vi "Cepstrum Analysis.vi"() -> ()   [LabVIEW 2023]
doc: "This example shows how to compute the real cepstrum of a univariate time series with the TSA Real Cepstrum VI, to compute the complex cepstrum of a univariate time series with the TSA Complex Cepstrum VI, and to reconstruct original time series with the TSA Inverse Complex Cepstrum VI. \n\n<b>Instructions:</b>\n1) Run this VI.\n2) Observe the real and complex cepstrum with different settings."
uses:
  <vilib>/addons/Time Series Analysis/Utilities.llb/TSA Data.ctl
  <vilib>/addons/Time Series Analysis/Correlation and Spectral Analysis.llb/TSA Complex Cepstrum (Waveform).vi
  <vilib>/addons/Time Series Analysis/Correlation and Spectral Analysis.llb/TSA Inverse Complex Cepstrum (Waveform).vi
  <vilib>/addons/Time Series Analysis/Correlation and Spectral Analysis.llb/TSA Real Cepstrum (Waveform).vi
  <vilib>/addons/_Advanced Signal Processing/NI_AdvSigProcTSA.lvlib
panel:
  in  "stop":bool
  in  "AR setting":cluster{"Method":u16, "AR Order":i32}={"Method"=0, "AR Order"=60} {"Method" items=["Forward-Backward", "Least-Squares", "Yule-Walker", "Burg-Lattice", "Geometric-Lattice"]}
  in  "Cepstrum bins":i32=-1
  in  "Window":u16(ring) items=["None ", "Hanning", "Hamming", "Blackman-Harris", "Exact Blackman", "Blackman", "Flat Top", "4 Term B-Harris ", "7 Term B-Harris", "Low Sidelobe"]
  in  "Method for Real Cepstrum":u16(ring) items=["FFT", "AR Model"]
  out "Complex Cepstrum":cluster{"t0":dbl, "dt":dbl, "C(t)":dbl[]}(graph)
  out "Vibration Series":waveform(dbl)[](graph)
  out "Real Cepstrum":cluster{"t0":dbl, "dt":dbl, "C(t)":dbl[]}(graph)
  # "Overview: Shows how to compute the real cepstrum of a univariate time series with the TSA Real Cepstrum VI, to compute the complex cepstrum of a univariate time series with  the TSA Complex Cepstrum VI, and to reconstruct original time series with the TSA Inverse Complex Cepstrum VI.\nRequirements: LabVIEW Full Development System, Advanced Signal Processing Toolkit\nInstructions: \n1. Run this VI.\n2. Observe the real and complex cepstrum with different settings.\n3. Click Stop to stop the VI."
  # "Cepstrum Settings"
  # "Settings for the FFT Method"
  # "Settings for the AR Model Method"
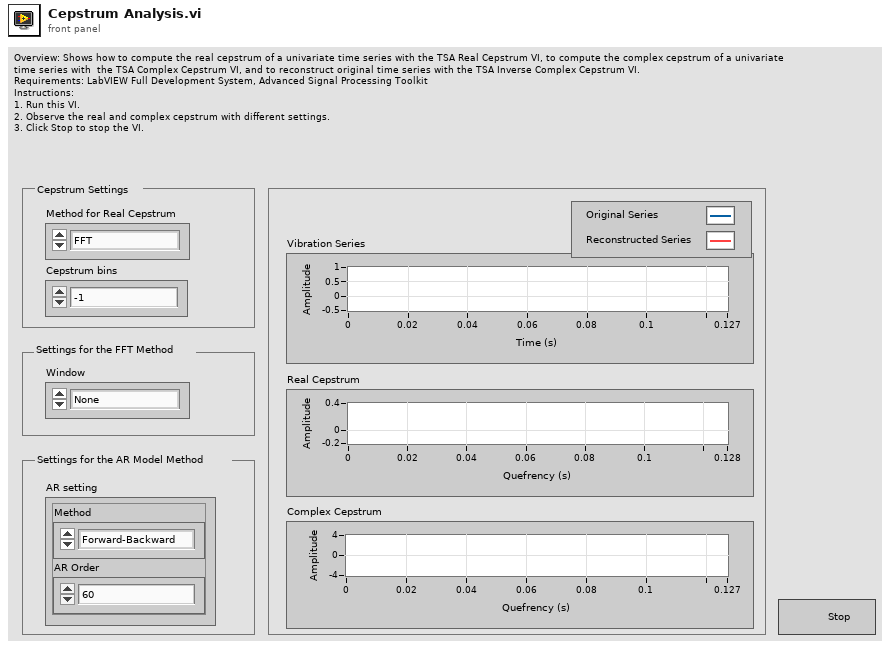
[diagram p1: front panel]
types:
  T1 = typedef "NI_AdvSigProcTSA.lvlib/TSA Data.ctl" = u16
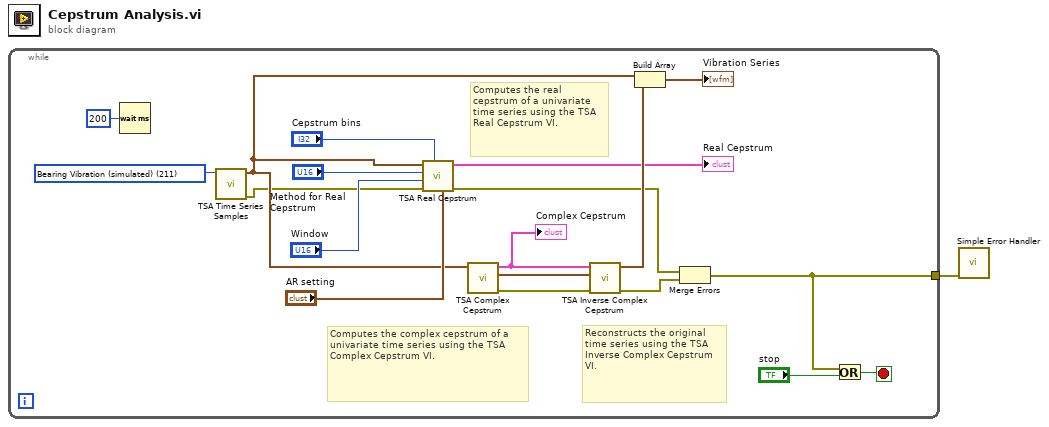
[diagram p0: block diagram]
diagram:
  n1 = while {
    tunnel: [w3] -> w1
    stop <- w7 stop-if-true
    w4 = T1 211 items=["Kobe Earthquake"=201, "EEG"=210, "Bearing Vibration (simulated)"=211, "Period Product Sales"=214, "Beam Vibration (nonlinear)"=217, "Beam Vibration (linear)"=218, "Signal With Echo"=219, "Engine Knocking"=220, "Power Line"=221, "-"=200, "Beam Deflections (multivariate)"=207, "Structure Vibration (multivariate)"=208, "Human MEG (multivariate)"=222] ("data")
    # "Reconstructs the original time series using the TSA Inverse Complex Cepstrum VI."
    # "Computes the complex cepstrum of a univariate time series using the TSA Complex Cepstrum VI."
    # "Computes the real cepstrum of a univariate time series using the TSA Real Cepstrum VI."
    n2 = Wait (ms)(milliseconds to wait=u32 200 ("millisecond multiple")) -> ()  [unwired: 1 out]
    n3 = call <vilib>:"TSA Time Series Samples.vi"("data"=w4) -> ("error out"=w2:errorcluster, "univariate time series"=w5:waveform(dbl))  [unwired: 1 in, 8 out]
    n4 = call-poly <vilib>:"TSA Real Cepstrum.vi"("AR setting"="AR setting", "cepstrum bins"="Cepstrum bins", "error in (no error)"=w2, "window"="Window", "method"="Method for Real Cepstrum", "Xt"=w5) -> ("error out"=w9:errorcluster, "cepstrum"=→"Real Cepstrum":cluster{"t0":dbl, "dt":dbl, "C(t)":dbl[]})  [unwired: 4 out]
    n5 = call-poly <vilib>:"TSA Complex Cepstrum.vi"("Xt"=w5) -> ("error out"=w20:errorcluster, "phase info"=w13:cluster{"DC":dbl, "Nyquist":dbl}, "cepstrum"=w16:cluster{"t0":dbl, "dt":dbl, "C(t)":dbl[]})  [unwired: 1 in, 7 out]
    "Complex Cepstrum" <- w16
    n6 = call-poly <vilib>:"TSA Inverse Complex Cepstrum.vi"("error in (no error)"=w20, "phase info"=w13, "cepstrum"=w16) -> ("error out"=w10:errorcluster, "Xt"=w18:waveform(dbl))  [unwired: 7 out]
    n7 = Build Array(w5, w18) -> (→"Vibration Series":waveform(dbl)[])
    n8 = Merge Errors(w9, w10) -> (w3:errorcluster)
    n9 = Or(x=w3, y="stop") -> (x .or. y?=w7:bool)
  }
  n10 = call <vilib>:"Simple Error Handler.vi"("error in (no error)"=w1) -> ()  [unwired: 1 in, 8 out]
